vi "WLAN_FrameAnalysis - Optimized - SIC.vi"(8 "error in (no error)":errorcluster, 10 "Decode SC":bool, 11 "input cluster":cluster{"t0":dbl, "dt":dbl, "Y":cdb[]}) -> (0 "error out":errorcluster, 1 "Constellation":cdb[](graph), 2 "Modulation parameter":T1, 3 "output bits":i8[](array[numeric]), 4 "Frequency offset":dbl, 5 "SIG valid?":bool)   [LabVIEW 2022 SP3]
panel:
  out "Constellation 2":cdb[](graph)
  out "x+y":dbl
  out "Frequency offset(LTF)":dbl
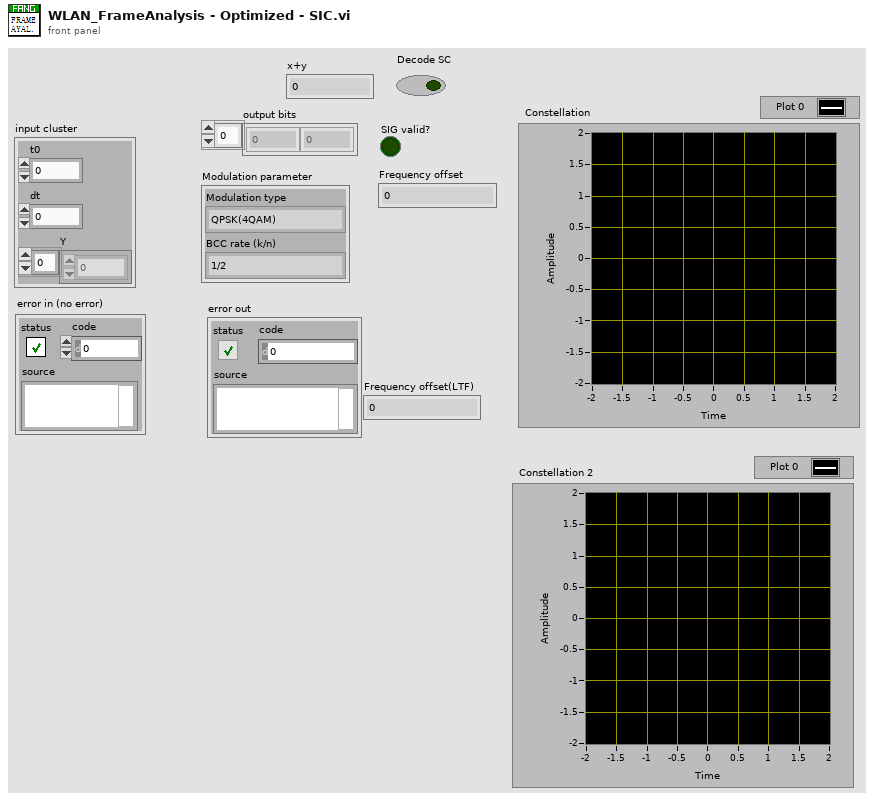
[diagram p1: front panel]
types:
  T1 = cluster{"Modulation type":enum16{"QPSK(4QAM)", "64QAM", "16QAM", "BPSK"}, "BCC rate (k/n)":enum16{"1/2", "2/3", "3/4"}}
  T2 = cluster{"Modulation type":enum16{"QPSK(4QAM)", "64QAM", "16QAM", "BPSK", "BPSK Vertical"}, "BCC rate (k/n)":enum16{"1/2", "2/3", "3/4"}}
  T3 = enum16{"QPSK(4QAM)", "64QAM", "16QAM", "BPSK", "BPSK Vertical"}
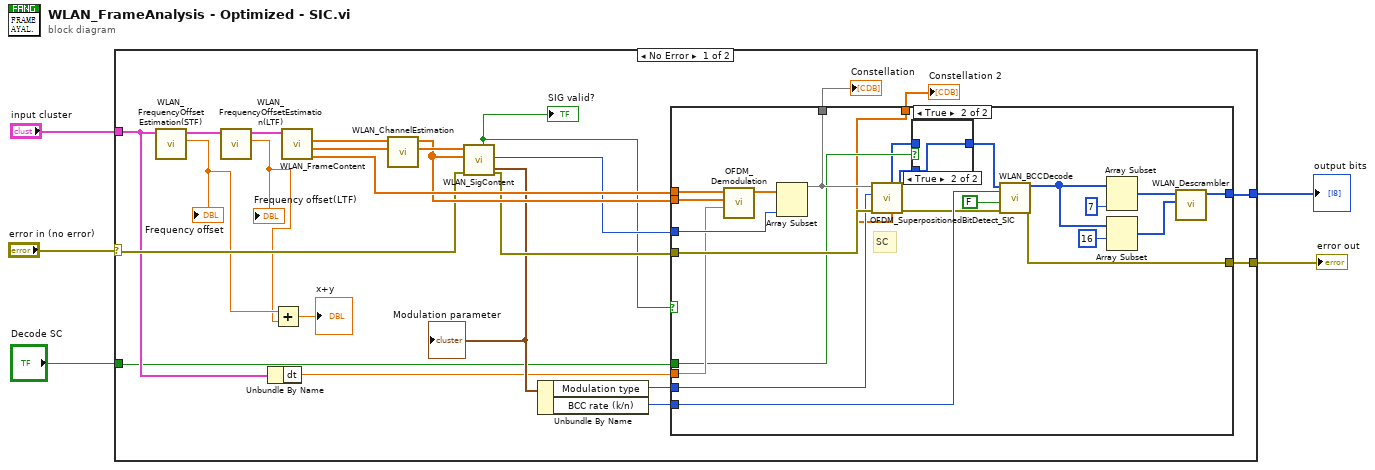
[diagram p0: block diagram]
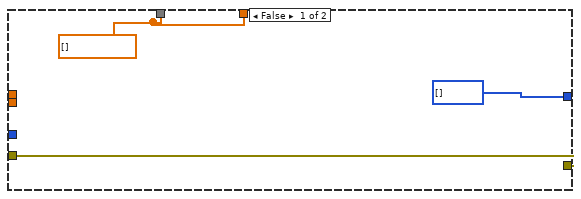
[diagram p2: hidden frame]
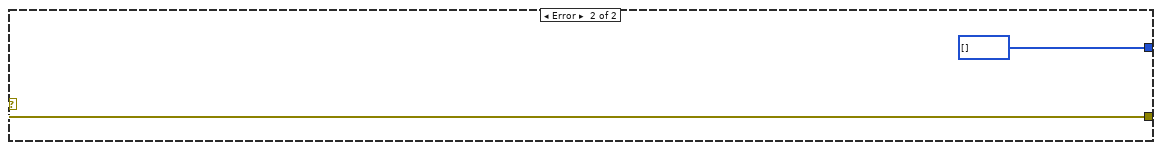
[diagram p4: hidden frame]
diagram:
  n1 = case shown="No Error" "error in (no error)" {
    selector: "error in (no error)" -> [w15 w57]
    tunnel: "input cluster" -> [w9 _]
    tunnel: [w22 w57] -> w4
    tunnel: [w21 i8[] [] ("scrambled bits")] -> w3
    tunnel: "Decode SC" -> [w7 _]
    frame No Error {
      n2 = call "WLAN_FrequencyOffsetEstimation(STF).vi"("output cluster"=w9) -> ("Frequency offset(STF)"=w13:dbl, "output cluster 2"=w14:cluster{"t0":dbl, "dt":dbl, "Y":cdb[]})  [unwired: 8 in]
      "Frequency offset" <- w13
      n3 = call "WLAN_FrequencyOffsetEstimation(LTF).vi"("input cluster"=w14) -> ("Frequency offset(LTF)"=w12:dbl, "output cluster"=w10:cluster{"t0":dbl, "dt":dbl, "Y":cdb[]})  [unwired: 9 in]
      "Frequency offset(LTF)" <- w12
      n4 = Unbundle By Name(w9) -> ("dt"=w8:dbl)
      n5 = Add(x=w13, y=w12) -> (x+y=→"x+y":dbl)
      n6 = call "WLAN_FrameContent.vi"("Input cluster"=w10) -> ("DATA"=w28:cdb[], "SIG"=w26:cdb[], "LTF"=w27:cdb[])  [unwired: 7 in, 1 out]
      n7 = call "WLAN_ChannelEstimation.vi"("LTF"=w27) -> ("Frequency estimation"=w25:cdb[])  [unwired: 10 in]
      n8 = call "WLAN_SigContent.vi"("error in (no error)"=w15, "Frequency channel estimation"=w25, "SIG"=w26) -> ("error out"=w24:errorcluster, "Symbol numbers"=w23:i32, "Modulation parameter"=w20:T2, "SIG valid?"=w16:bool)  [unwired: 3 in, 2 out]
      "Modulation parameter" <- w20
      "SIG valid?" <- w16
      n9 = Unbundle By Name(w20) -> ("Modulation type"=w19:T3, "BCC rate (k/n)"=w18:enum16{"1/2", "2/3", "3/4"})
      n10 = case shown="True" w16 {
        tunnel: w28 -> [_ w54]
        tunnel: [w31 w46] -> w22
        tunnel: w25 -> [_ w52]
        tunnel: w24 -> [w31 w51]
        tunnel: w23 -> [_ w50]
        tunnel: w19 -> [_ w49]
        tunnel: [i8[] [] ("scrambled bits") w38] -> w21
        tunnel: w18 -> [_ w48]
        tunnel: [w29 w40] -> w17
        tunnel: w8 -> [_ w37]
        tunnel: w7 -> [_ w36]
        tunnel: [w29 w32] -> w6
        frame False {
          w29 = cdb[] []
        }
        frame True {
          # "SC"
          n11 = call "OFDM_Demodulation.vi"("sampling period"=w37, "Frequency channel estimation"=w52, "Input sequence"=w54) -> ("Output sequence"=w53:cdb[])  [unwired: 7 in, 1 out]
          n12 = Array Subset(array=w53, length=w50) -> (w40:cdb[])  [unwired: 1 in]
          n13 = call "OFDM_SuperpositionedBitDetect_SIC.vi"("Input symbols"=w40, "Modulation type"=w49, "error in (no error)"=w51) -> ("Base Bits"=w35:i8[], "SC Symbols"=w32:cdb[], "SC Bits"=w34:i8[], "error out"=w47:errorcluster)  [unwired: 4 in]
          n14 = case shown="True" w36 {
            tunnel: w35 -> [w55 _]
            tunnel: w34 -> [_ w56]
            tunnel: [w55 w56] -> w33
            frame False {
            }
            frame True {
            }
          }
          n15 = call "WLAN_BCCDecode.vi"("error in (no error)"=w47, "need add zeros?"=FALSE, "BCC rate (k/n)"=w48, "input bit stream"=w33) -> ("error out"=w46:errorcluster, "output bit stream"=w39:i8[])  [unwired: 6 in]
          n16 = Array Subset(array=w39, length=7) -> (w42:i8[])  [unwired: 1 in]
          n17 = Array Subset(array=w39, index=16) -> (w43:i8[])  [unwired: 1 in]
          n18 = call "WLAN_Descrambler.vi"("scrambler initial bits"=w42, "data bits"=w43) -> ("scrambled bits"=w38:i8[])  [unwired: 7 in]
        }
      }
      "Constellation" <- w17
      "Constellation 2" <- w6
    }
    frame Error {
    }
  }
  "error out" <- w4
  "output bits" <- w3
